vi "Read.vi"(4 "Where":string, 6 "commandTimeout":i32, 8 "error in (no error)":errorcluster, 9 "DynamicParameters":refnum<class "DynamicParameters.lvclass">, 10 "TableName":string, 11 "SqlMapper in":refnum<class "SqlMapper.lvclass">) -> (0 "error out":errorcluster, 2 "Value":variant, 3 "SqlMapper out":refnum<class "SqlMapper.lvclass">)   [LabVIEW 2020, in "ORM.lvlib" / "SqlMapper.lvclass"]
uses:
  SqlMapper.lvclass
  DynamicParameters/DynamicParameters.lvclass
  SqlMapper.lvclass/SqlMapper.ctl
  DbConnection/DbConnection.lvclass
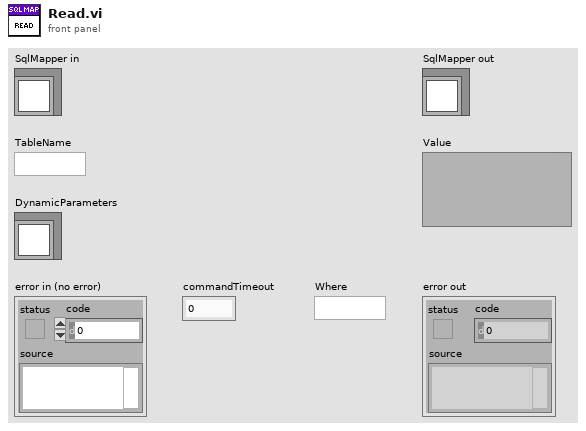
[diagram p1: front panel]
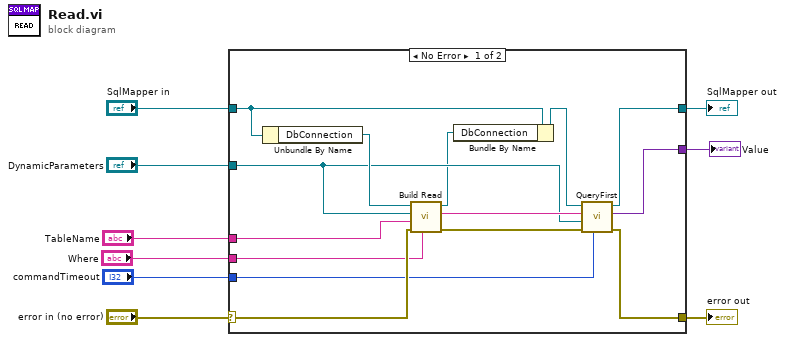
[diagram p0: block diagram]
diagram:
  n1 = case shown="No Error" "error in (no error)" {
    selector: "error in (no error)" -> [w18 w25]
    tunnel: [w13 w25] -> w8
    tunnel: [w15 w24] -> w6
    tunnel: "SqlMapper in" -> [w21 w24]
    tunnel: "DynamicParameters" -> [w19 _]
    tunnel: "TableName" -> [w22 _]
    tunnel: "commandTimeout" -> [w16 _]
    tunnel: [w14 _] -> w2
    tunnel: "Where" -> [w10 _]
    frame No Error {
      n2 = Unbundle By Name(w21) -> ("DbConnection"=w23:refnum<class "DbConnection.lvclass">)
      n3 = call-dynamic "Build Read.vi"("Where"=w10, "error in (no error)"=w18, "tableName"=w22, "DynamicParameters in"=w19, "DbConnection in"=w23) -> ("error out"=w17:errorcluster, "Query"=w20:string, "DbConnection out"=w11:refnum<class "DbConnection.lvclass">)  [unwired: 4 in]
      n4 = Bundle By Name(cluster=w21, "DbConnection"=w11) -> (w12:refnum<class "SqlMapper.lvclass">)
      n5 = call-dynamic "QueryFirst.vi"("commandTimeout in"=w16, "error in (no error)"=w17, "DynamicParameters in"=w19, "sql"=w20, "SqlMapper in"=w12) -> ("error out"=w13:errorcluster, "Value"=w14:variant, "SqlMapper out"=w15:refnum<class "SqlMapper.lvclass">)  [unwired: 4 in]
    }
    frame Error {
    }
  }
  "error out" <- w8
  "SqlMapper out" <- w6
  "Value" <- w2
